vi "Confirm Disable Buffering (SubVI).vi"(8 "error constant 2":errorcluster, 11 "Disable Buffering in":bool) -> (0 "error constant":errorcluster, 3 "Disable Buffering out":bool)   [LabVIEW 2023]
panel:
  in  "Continue":bool
  in  "Stop":bool caption="y"
  # "If this is not on, it's likely normal\nPlease consult NI documentation for including this optimization"
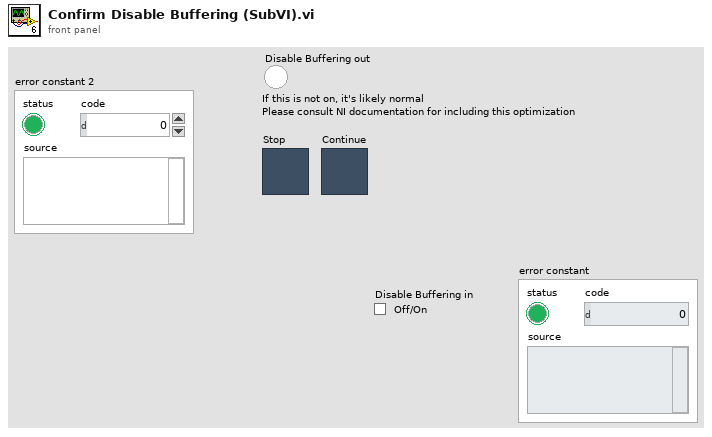
[diagram p1: front panel]
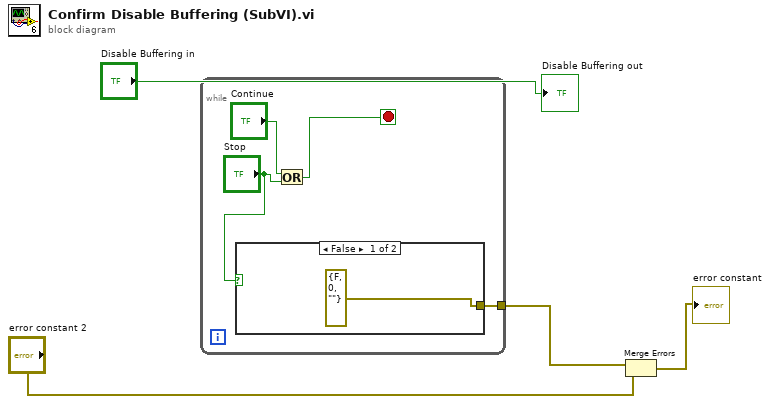
[diagram p0: block diagram]
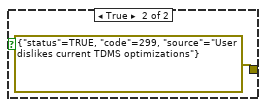
[diagram p2: hidden frame]
diagram:
  n1 = while {
    tunnel: [w6] -> w3
    stop <- w8 stop-if-true
    n2 = case shown="False" "Stop" {
      tunnel: [errorcluster {"status"=FALSE, "code"=0, "source"=""} ("error constant") errorcluster {"status"=TRUE, "code"=299, "source"="User dislikes current TDMS optimizations"} ("error constant")] -> w6
      frame False {
      }
      frame True {
      }
    }
    n3 = Or(x="Continue", y="Stop") -> (x .or. y?=w8:bool)
  }
  n4 = Merge Errors(w3, "error constant 2") -> (→"error constant":errorcluster)
  "Disable Buffering out" <- "Disable Buffering in"
